vi "InsertStep.vi"(0 "Script in":T3, 5 "new element/subarray":T1={"Direction"=enum."Chamber", "Pressure MPa"=0.0, "Time s"=0.0, "Delta alarm MPa"=0.0, "Delta warning MPa"=0.0}, 7 "index in":i32) -> (4 "Script out":T3, 6 "index out":i32)   [LabVIEW 2019]
uses:
  TypeDef/Script.ctl
  TypeDef/Step.ctl
  TypeDef/Direction.ctl
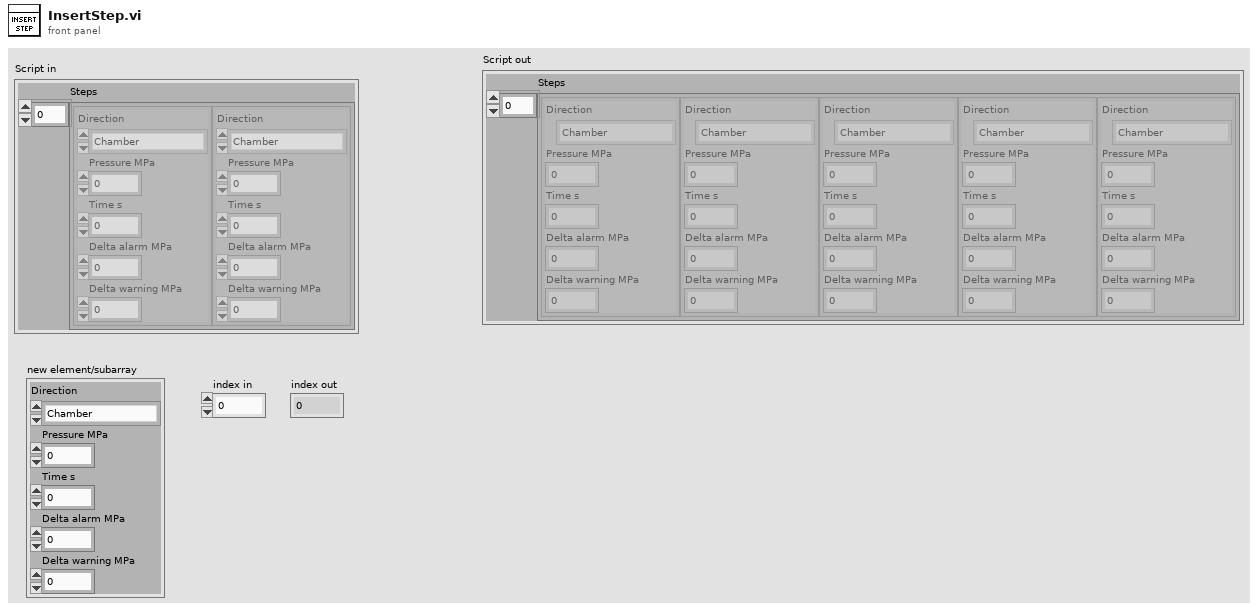
[diagram p1: front panel]
types:
  T1 = typedef "Step.ctl" = cluster{"Direction":T2, "Pressure MPa":dbl, "Time s":dbl, "Delta alarm MPa":dbl, "Delta warning MPa":dbl}
  T2 = typedef "Direction.ctl" = enum16{"None", "Chamber", "DUT"}
  T3 = typedef "Script.ctl" = cluster{"Steps":T1[]}
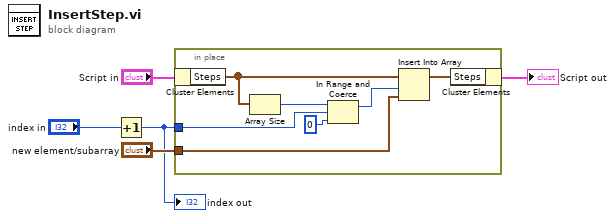
[diagram p0: block diagram]
diagram:
  n1 = Increment(x="index in") -> (x+1=w1:i32)
  "index out" <- w1
  n2 = in-place {
    in-place-border: "new element/subarray" -> [w11]
    in-place-border: w1 -> [w6]
    n3 = in-place-cluster #1("Script in") -> ("Steps"=w9:T1[])
    n4 = Array Size(array=w9) -> (size(s)=w8:i32)
    n5 = In Range and Coerce(upper limit=w8, x=w6, lower limit=0) -> (coerced(x)=w7:i32)  [unwired: 1 out]
    n6 = Insert Into Array(array=w9, index=w7, new element=w11) -> (w12:T1[])
    n7 = in-place-cluster #1("Steps"=w12) -> (→"Script out":T3)
  }
